vi "Render.vi"   [LabVIEW 2018, in "Toolkit.lvlib" / "Render.lvclass"]
uses:
  Render.lvclass
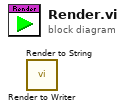
[diagram p0: block diagram]
diagram:
  n1 = call "Render to Writer.vi"() -> ()  [unwired: 9 in, 3 out]
  n2 = call "Render to String.vi"() -> ()  [unwired: 9 in, 3 out]
